vi "Vision Processing.vi"(4 "error in (no error)":errorcluster, 6 "CameraDevRef":T1) -> ()   [LabVIEW 2011]
uses:
  <vilib>/Rock Robotics/WPI/Camera/WPI_CameraDevRef.ctl
  Robot Global Data.vi
  <vilib>/vision/NI_Vision_Development_Module.lvlib
panel:
  in  "Max Distance for 1 hoop":dbl=8.0
  out "Raw Turret":dbl
  in  "Run Calculations":bool
  out "Target X Coord":dbl
  out "Target Distance":dbl
  out "Target Y Coord":dbl
  out "Distance Array":dbl[](array[numeric])
  in  "Scaler":dbl=0.85
  in  "Lower Speed Limit":dbl=0.05
  out "Number of Rectangles Visible":dbl
  out "Y Position Array":dbl[](array[numeric])
  out "X Position Array":dbl[](array[numeric])
  in  "View":bool
  out "Target Info":T2(array[cluster])
  in  "Area Size Limit":i32=444
  in  "Particle Count Limit":i32=8
  in  "Score Limits":T3={"Rect Coverage"=76.0, "Aspect Ratio"=40.0, "X Edge Strength"=40.0, "Y Edge Strength"=60.0}
  in  "Processing":enum32{"Color", "Intensity", "Intensity Open"}(tab)=enum."Intensity"
  in  "Luminance":i32=255
  in  "Saturation":i32=255
  in  "Hue":i32(knob)=65 scale=0.0..255.0
  in  "Margins":cluster{"Hue":i32, "Sat":i32, "Lum":i32}={"Hue"=20, "Sat"=27, "Lum"=30} {"Sat" scale=0.0..40.0; "Lum" scale=0.0..40.0; "Hue" scale=0.0..40.0}
  in  "Range":cluster{"Lower value":sgl, "Upper value":sgl}={"Lower value"=107.17391, "Upper value"=255.0} {"Lower value" scale=0.0..255.0; "Upper value" scale=0.0..255.0}
  in  "Range":cluster{"Lower value":sgl, "Upper value":sgl}={"Lower value"=123.804344, "Upper value"=255.0} {"Lower value" scale=0.0..255.0; "Upper value" scale=0.0..255.0}
  in  "View":bool
  out "Processed Image":T4(plugin-control)
  out "Original Image":T4(plugin-control)
  # "Instructions:\nProcessing the reflective tape that is illuminated by a ring light can be based\non color or light intensity.\nParticles within the image are scored by rectangle coverage, aspect ratio, and\nfor being hollow with a bold edge. A particle is considered a target if all scores\nare above the score limits. Particles can be annotated -- surrounded by\na rectangle and scores drawn to the left .\nTo control the number of particles being scored, use the count limit and the size\nlimit."
  # "(in)"
  # "To debug, Enable using the View button.\nFor color processing, you can click in the image to select the color for processing."
  # "Enable by clicking the View button.\nGreen scores are above the limit, orange are below. Inner/outer rect\nindicates all passed."
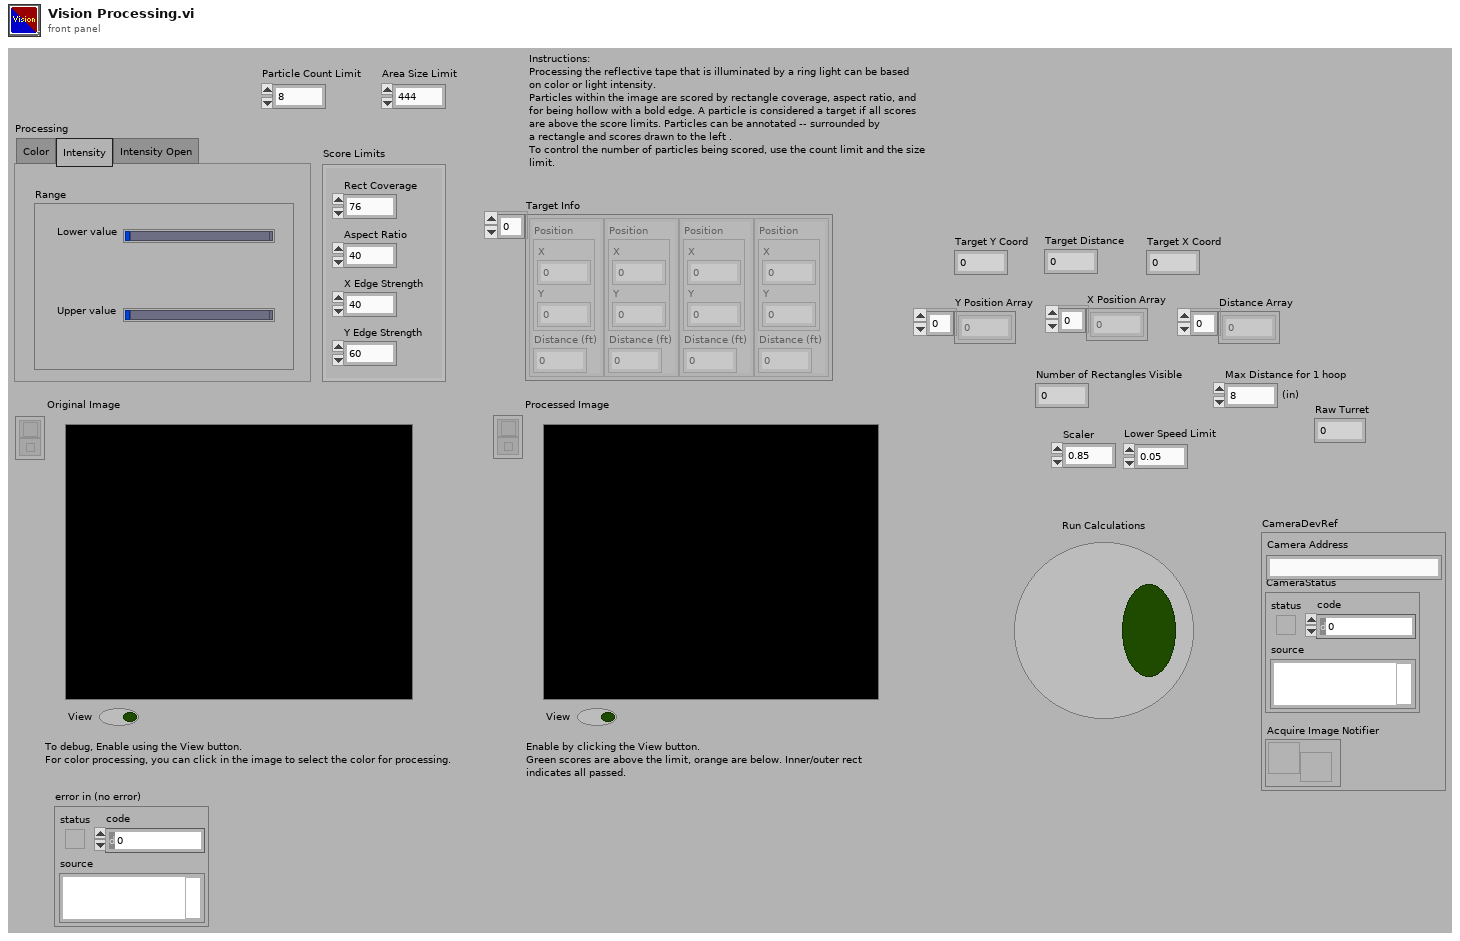
[diagram p1: front panel]
types:
  T1 = typedef "WPI_CameraDevRef.ctl" = cluster{"Camera Address":string, "CameraStatus":errorcluster, "Acquire Image Notifier":refnum<notifier>}
  T2 = cluster{"Position":cluster{"X":dbl, "Y":dbl}, "Distance (ft)":dbl}[]
  T3 = cluster{"Rect Coverage":dbl, "Aspect Ratio":dbl, "X Edge Strength":dbl, "Y Edge Strength":dbl}
  T4 = typedef "IMAQ Image.ctl" = refnum<image>
  T5 = typedef "Image Type" = u32
  T6 = enum32{"AutoM", "Close", "Dilate", "Erode", "Gradient", "Gradient out", "Gradient in", "Hit miss", "Open", "PClose", "POpen", "Thick", "Thin"}
  T7 = typedef "WPI_CameraImageSize.ctl" = enum16{"640x480", "320x240", "160x120"}
  T8 = cluster{"fps":i32, "compression":i32, "Image Size":T7}
  T9 = cluster{cluster{"Left":dbl, "Top":dbl, "Right":dbl, "Bottom":dbl}, dbl[]}[]
  T10 = cluster{"Left":dbl, "Top":dbl, "Right":dbl, "Bottom":dbl}
  T11 = cluster{"Target Center (-1 to 1)":cluster{"X":dbl, "Y":dbl}, "Distance (ft)":dbl}
  T12 = cluster{"Target Center (-1 to 1)":cluster{"X":dbl, "Y":dbl}, "Distance (ft)":dbl}[]
  T13 = typedef "WPI_JoystickDevRef.ctl" = cluster{"Device":T14}
  T14 = typedef "WPI_JoystickDeviceEnum.ctl" = enum16{"USB 1", "USB 2", "USB 3", "USB 4", "Kinect 1", "Kinect 2"}
  T15 = typedef "WPI_JoystickButtonState.ctl" = cluster{"Button 1":bool, "Button 2":bool, "Button 3":bool, "Button 4":bool, "Button 5":bool, "Button 6":bool, "Button 7":bool, "Button 8":bool, "Button 9":bool, "Button 10":bool, "Button 11":bool, "Button 12":bool}
  T16 = cluster{"axis 1 (x)":dbl, "axis 2 (y)":dbl, "axis 3 (throttle)":dbl, "axis 4":dbl, "axis 5":dbl, "axis 6":dbl}
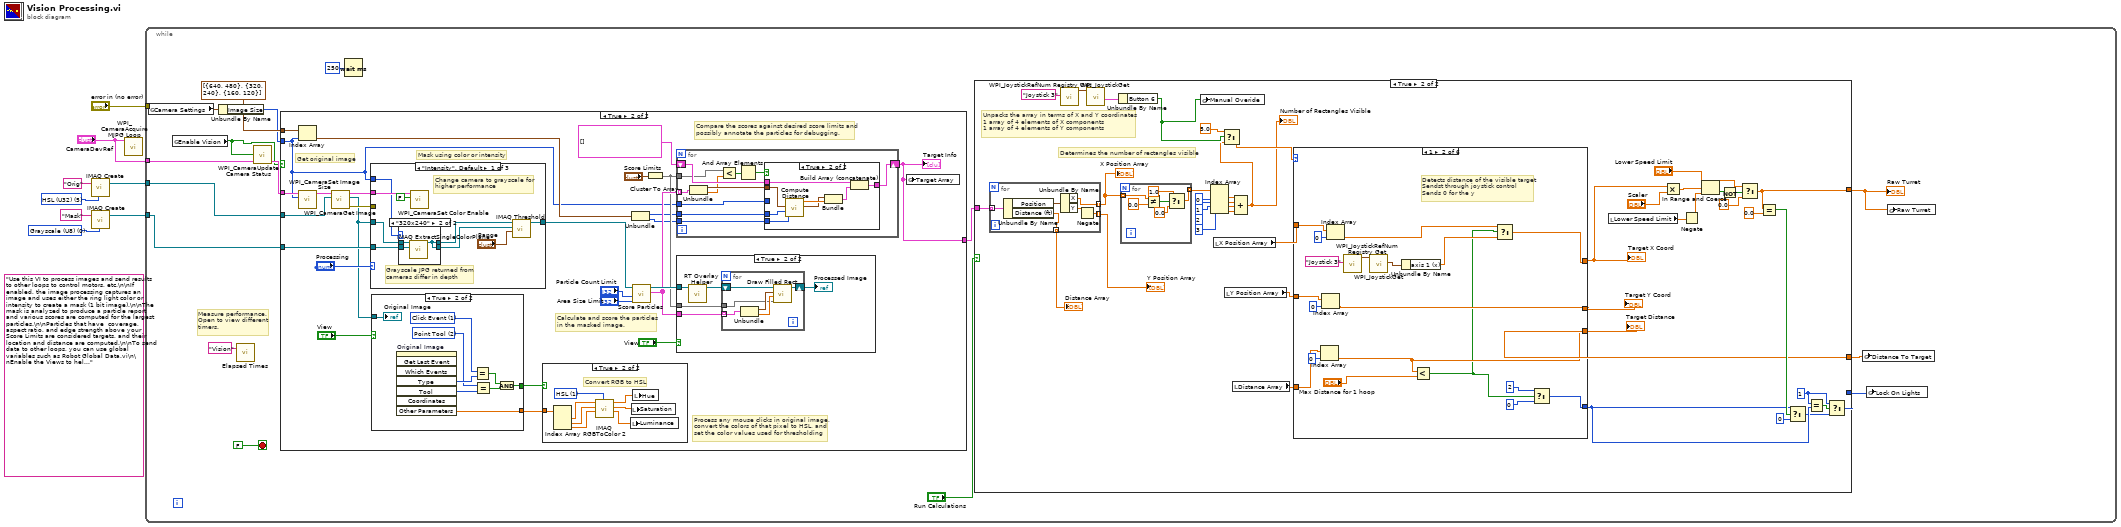
[diagram p0: block diagram]
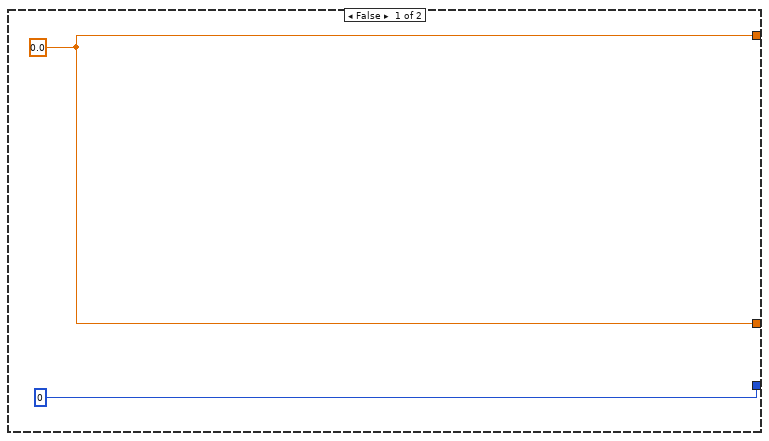
[diagram p2: hidden frame]
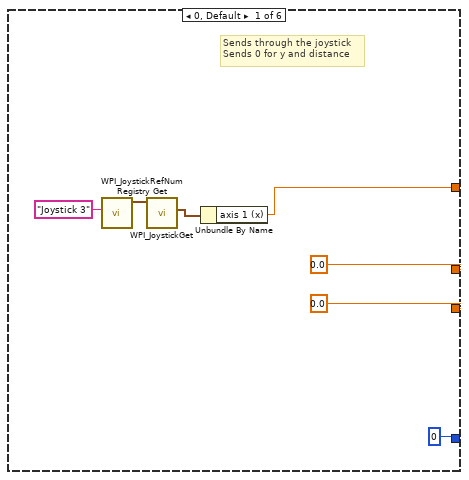
[diagram p3: hidden frame]
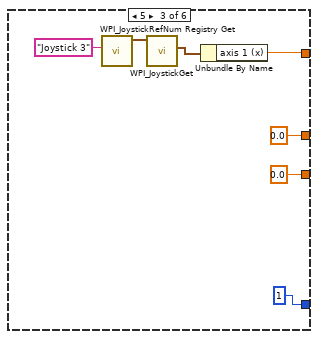
[diagram p4: hidden frame]
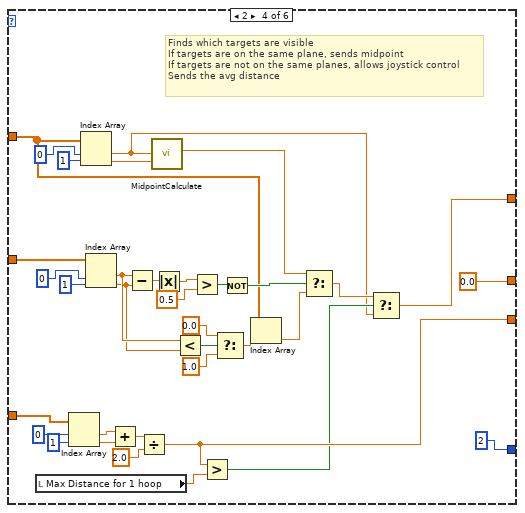
[diagram p5: hidden frame]
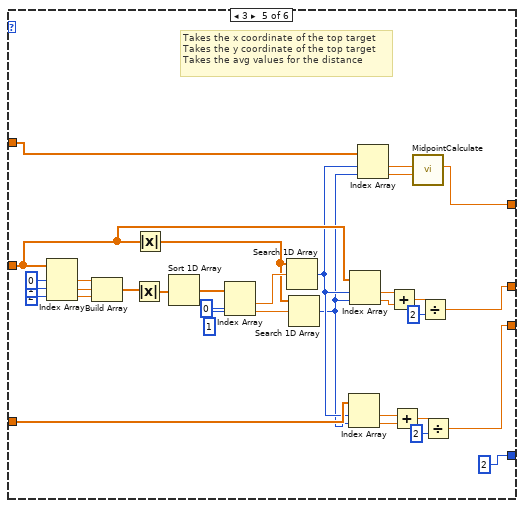
[diagram p6: hidden frame]
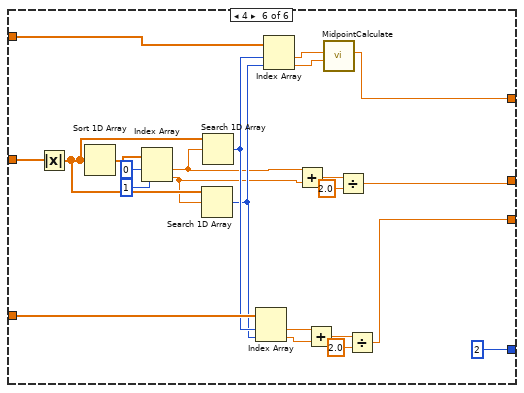
[diagram p7: hidden frame]
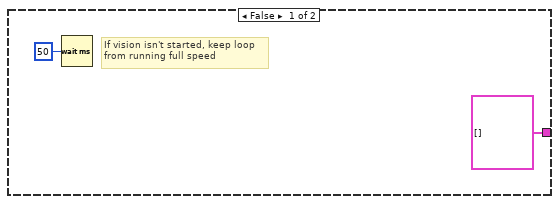
[diagram p8: hidden frame]
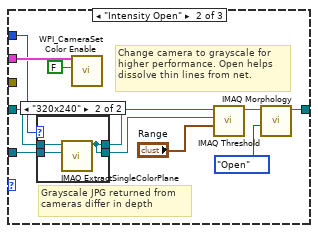
[diagram p11: hidden frame]
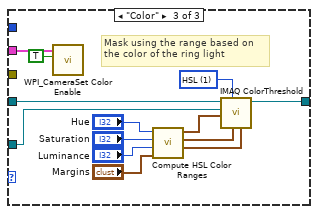
[diagram p13: hidden frame]
diagram:
  w3 = T5 0 items=["Grayscale (U8)", "Grayscale (I16)", "Grayscale (SGL)", "Complex (CSG)", "RGB (U32)", "HSL (U32)", "RGB (U64)", "Grayscale (U16)"] ("Image Type")
  (unwired) "Use this VI to process images and send results to other loops to control motors, etc.\n\nIf enabled, the image processing captures an image and uses either the ring light color or intensity to create a mask (1 bit image).\n\nThe mask is analyzed to produce a particle report and various scores are computed for the largest particles.\n\nParticles that have  coverage, aspect ratio, and edge strength above your Score Limits are considered targets, and their location and distance are computed.\n\nTo send data to other loops, you can use global variables such as Robot Global Data.vi\n\nEnable the Views to help debug color settings. Disable the View to speed up processing."
  w7 = T5 5 items=["Grayscale (U8)", "Grayscale (I16)", "Grayscale (SGL)", "Complex (CSG)", "RGB (U32)", "HSL (U32)", "RGB (U64)", "Grayscale (U16)"] ("Image Type")
  n1 = call "IMAQ Create"("Image Name"="Orig", "Image Type"=w7) -> ("New Image"=w6:T4)  [unwired: 2 in, 2 out]
  n2 = call "IMAQ Create"("Image Name"="Mask", "Image Type"=w3) -> ("New Image"=w1:T4)  [unwired: 2 in, 2 out]
  n3 = call <vilib>:"WPI_CameraAcquire MJPG Loop.vi"("CameraDevRef"="CameraDevRef") -> ()  [unwired: 11 in]
  n4 = while {
    tunnel: w6 -> [w23]
    tunnel: "CameraDevRef" -> [w22]
    tunnel: "error in (no error)" -> [_]
    tunnel: w1 -> [w18]
    stop <- FALSE stop-if-true
    # "Measure performance.\nOpen to view different\ntimers."
    n5 = global read "Robot Global Data.vi" "Camera Settings"() -> (w16:T8)
    n6 = global read "Robot Global Data.vi" "Enable Vision"() -> (w20:bool)
    n7 = Unbundle By Name(w16) -> ("Image Size"=w15:T7)
    n8 = call "Elapsed Times.vi"("Call Name"="Vision") -> ()  [unwired: 2 in, 1 out]
    n9 = call <vilib>:"WPI_CameraUpdate Camera Status.vi"("CameraDevRef In"=w22, "Enable Vision"=w20) -> ("CameraDevRef Out"=w21:T1)  [unwired: 3 in]
    n10 = case shown="True" w20 {
      tunnel: w23 -> [_ w224]
      tunnel: w21 -> [_ w220]
      tunnel: w18 -> [_ w211]
      tunnel: cluster{i32, i32}[] [{640, 480}, {320, 240}, {160, 120}] -> [_ w215]
      tunnel: w15 -> [_ w208]
      tunnel: [T2 [] w209] -> w14
      frame False {
        # "If vision isn't started, keep loop\nfrom running full speed"
        n11 = Wait (ms)(milliseconds to wait=u32 50) -> ()  [unwired: 1 out]
      }
      frame True {
        # "Compare the scores against desired score limits and\npossibly annotate the particles for debugging."
        # "Process any mouse clicks in original image,\nconvert the colors of that pixel to HSL, and\nset the color values used for thresholding"
        # "Calculate and score the particles\nin the masked image."
        # "Mask using color or intensity"
        # "Get original image"
        n12 = call <vilib>:"WPI_CameraSet Image Size.vi"("Image Size"=w208, "CameraDevRef"=w220) -> ("CameraDevRef Out"=w221:T1)  [unwired: 8 in, 1 out]
        n13 = Index Array(array=w215, index=w208) -> (element=w212:cluster{i32, i32})
        n14 = call <vilib>:"WPI_CameraGet Image.vi"("Image"=w224, "CameraDevRef"=w221) -> ("error out"=w222:errorcluster, "Image Out"=w210:T4, "CameraDevRef Out"=w223:T1)  [unwired: 7 in]
        n15 = case shown="\"Intensity\", Default" "Processing" {
          tunnel: w210 -> [w246 w258 w284]
          tunnel: [w249 w263 w283] -> w218
          tunnel: w223 -> [w247 w261 w274]
          tunnel: w222 -> [_ _ _]
          tunnel: w211 -> [w245 w259 w272]
          tunnel: w208 -> [w244 w260 _]
          frame "Intensity", Default {
            # "Grayscale JPG returned from\ncameras differ in depth"
            # "Change camera to grayscale for\nhigher performance"
            n16 = case shown="\"320x240\"" w244 {
              tunnel: w246 -> [w252 w255]
              tunnel: w245 -> [w251 w254]
              tunnel: [w252 w253] -> w243
              tunnel: [w251 w253] -> w242
              frame "640x480", Default {
              }
              frame "320x240" {
                n17 = call "IMAQ ExtractSingleColorPlane"("Image Dst"=w254, "Image Src"=w255) -> ("Image Dst Out"=w253:T4)  [unwired: 8 in, 1 out]
              }
            }
            n18 = call <vilib>:"WPI_CameraSet Color Enable.vi"("Color Enabled"=FALSE, "CameraDevRef"=w247) -> ()  [unwired: 8 in, 2 out]
            n19 = call "IMAQ Threshold"("Range"="Range", "Image Dst"=w242, "Image Src"=w243) -> ("Image Dst Out"=w249:T4)  [unwired: 3 in, 5 out]
          }
          frame "Intensity Open" {
            # "Grayscale JPG returned from\ncameras differ in depth"
            # "Change camera to grayscale for\nhigher performance. Open helps\ndissolve thin lines from net."
            n20 = case shown="\"320x240\"" w260 {
              tunnel: w258 -> [w268 w271]
              tunnel: w259 -> [w267 w270]
              tunnel: [w268 w269] -> w257
              tunnel: [w267 w269] -> w256
              frame "640x480", Default {
              }
              frame "320x240" {
                n21 = call "IMAQ ExtractSingleColorPlane"("Image Dst"=w270, "Image Src"=w271) -> ("Image Dst Out"=w269:T4)  [unwired: 8 in, 1 out]
              }
            }
            n22 = call <vilib>:"WPI_CameraSet Color Enable.vi"("Color Enabled"=FALSE, "CameraDevRef"=w261) -> ()  [unwired: 8 in, 2 out]
            n23 = call "IMAQ Threshold"("Range"="Range", "Image Dst"=w256, "Image Src"=w257) -> ("Image Dst Out"=w264:T4)  [unwired: 3 in, 5 out]
            n24 = call "IMAQ Morphology"("Operation"=T6."Open", "Image Src"=w264) -> ("Image Dst Out"=w263:T4)  [unwired: 8 in, 1 out]
          }
          frame "Color" {
            w282 = u16 1 items=["RGB", "HSL", "HSV", "HSI"] ("Color Mode")
            # "Mask using the range based on\nthe color of the ring light"
            n25 = call <vilib>:"WPI_CameraSet Color Enable.vi"("Color Enabled"=TRUE, "CameraDevRef"=w274) -> ()  [unwired: 8 in, 2 out]
            n26 = call "Compute HSL Color Ranges.vi"("Margins"="Margins", "Luminance"="Luminance", "Saturation"="Saturation", "Hue"="Hue") -> ("Lum Range"=w279:cluster{i32, i32}, "Sat Range"=w280:cluster{i32, i32}, "Hue Range"=w281:cluster{i32, i32})  [unwired: 5 in]
            n27 = call "IMAQ ColorThreshold"("Blue or Luma or Val or Inten Range"=w279, "Green or Sat Range"=w280, "Color Mode"=w282, "Red or Hue Range"=w281, "Image Dst"=w272, "Image Src"=w284) -> ("Image Dst Out"=w283:T4)  [unwired: 4 in, 1 out]
          }
        }
        n28 = case shown="True" "View" {
          tunnel: w210 -> [_ w304]
          tunnel: [_ w299] -> w217
          tunnel: [_ w296] -> w216
          frame False {
          }
          frame True {
            w297 = 2 items=["None", "Selection Tool", "Point Tool", "Line Tool", "Rectangle Tool", "Oval Tool", "Polygon Tool", "ClosedFreehandTool", "Annulus Tool", "Rotated Rectangle Tool", "Zoom Tool", "Pan Tool", "Polyline Tool", "Freehand Tool"] ("Tool")
            w298 = 1 items=["No Event"=0, "Click Event"=1, "Draw Event"=2, "Size Event"=4, "Scroll Event"=5, "Double Click Event"=8] ("Type")
            n29 = invoke on="Original Image" class="ImageControl" method="Get Last Event"() -> ("Type"=w300:i32, "Tool"=w303:i32, "Other Parameters"=w296:sgl[])  [unwired: 8 in, 5 out]
            n30 = Equal?(x=w298, y=w300) -> (x = y?=w301:bool)
            n31 = Equal?(x=w297, y=w303) -> (x = y?=w302:bool)
            n32 = And(x=w301, y=w302) -> (x .and. y?=w299:bool)
            "Original Image" <- w304
          }
        }
        n33 = case shown="True" w217 {
          tunnel: w216 -> [_ w241]
          frame False {
          }
          frame True {
            w240 = u16 1 items=["RGB", "HSL", "HSV", "HSI", "CIE L*a*b*", "CIE XYZ"] ("Color Mode")
            # "Convert RGB to HSL"
            n34 = Index Array(array=w241) -> (element #1=w239:sgl, element #2=w237:sgl, element #3=w235:sgl)  [unwired: 3 in]
            n35 = call "IMAQ RGBToColor 2"("Color Mode"=w240, "Blue value"=w235, "Green value"=w237, "Red value"=w239) -> ("Blue or Luma or Val or Inten or Z or b*value"=w234:dbl, "Green or Sat or Y or a* value"=w236:dbl, "Red or Hue or X or L* value"=w238:dbl)  [unwired: 4 in, 1 out]
            n36 = local write "Luminance"(w234) -> ()
            n37 = local write "Saturation"(w236) -> ()
            n38 = local write "Hue"(w238) -> ()
          }
        }
        n39 = Unbundle(w212) -> (w214:i32, w213:i32)
        n40 = call "Score Particles.vi"("Area Size Limit"="Area Size Limit", "Particle Count Limit"="Particle Count Limit", "Image Refnum in"=w218) -> ("Scored Particle Info"=w229:T9, "Image Refnum out"=w232:T4)  [unwired: 7 in]
        n41 = Cluster To Array(cluster="Score Limits") -> (array=w227:dbl[])
        n42 = for {
          shift-right: [w314] -> w209
          shift-left: T2 [] -> [w315]
          tunnel: w214 -> [w313]
          tunnel: w229 -> [w311] mode=indexing
          tunnel: w227 -> [w306]
          tunnel: w208 -> [w310]
          tunnel: w213 -> [w305]
          n43 = Unbundle(w311) -> (w312:T10, w307:dbl[])
          n44 = Less?(x=w306, y=w307) -> (x < y?=w309:bool[])
          n45 = And Array Elements(Boolean array=w309) -> (logical AND=w308:bool)
          n46 = case shown="True" w308 {
            tunnel: w315 -> [w316 w324]
            tunnel: [w316 w323] -> w314
            tunnel: w312 -> [_ w319]
            tunnel: w313 -> [_ w321]
            tunnel: w310 -> [_ _]
            tunnel: w305 -> [_ w318]
            frame False {
            }
            frame True {
              n47 = call "Compute Distance.vi"("Y Image Resolution"=w318, "X Image Resolution"=w321, "Bounding Box"=w319) -> ("Target Center (-1 to 1)"=w317:cluster{"X":dbl, "Y":dbl}, "Distance (ft)"=w320:dbl)  [unwired: 7 in]
              n48 = Bundle("Target Center (-1 to 1)"=w317, "Distance (ft)"=w320) -> (w322:T11)  [unwired: 1 in]
              n49 = Build Array (concatenate)(w324, w322) -> (w323:T12)
            }
          }
        }
        "Target Info" <- w209
        n50 = case shown="True" "View" {
          tunnel: w232 -> [_ w286]
          tunnel: w229 -> [_ w288]
          tunnel: w227 -> [_ w287]
          frame False {
          }
          frame True {
            n51 = call "RT Overlay Helper.vi"("Refnum in"=w286) -> ("Refnum out"=w289:T4)  [unwired: 10 in]
            n52 = for {
              shift-right: [w294] -> w285
              shift-left: w289 -> [w295]
              tunnel: w288 -> [w291] mode=indexing
              tunnel: w287 -> [w290]
              n53 = Unbundle(w291) -> (w292:T10, w293:dbl[])
              n54 = call "Draw Filled Rect.vi"("Limits"=w290, "Scores"=w293, "Bounding Box"=w292, "image in"=w295) -> ("image out"=w294:T4)  [unwired: 7 in]
            }
            "Processed Image" <- w285
          }
        }
        n55 = global write "Robot Global Data.vi" "Target Array"(w209) -> ()
      }
    }
    n56 = Wait (ms)(milliseconds to wait=u32 250) -> ()  [unwired: 1 out]
    n57 = case shown="True" "Run Calculations" {
      tunnel: w14 -> [_ w42]
      tunnel: [w25 w36] -> w11
      tunnel: [0 ("f") w33] -> w10
      tunnel: [w25 w28] -> w9
      frame False {
        w25 = 0.0 ("f")
      }
      frame True {
        w34 = 1 ("y")
        # "Determines the number of rectangles visible"
        # "Unpacks the array in terms of X and Y coordinates\n1 array of 4 elements of X components\n1 array of 4 elements of Y components"
        n58 = for {
          tunnel: [w203] -> w43 mode=indexing
          tunnel: [w204] -> w53 mode=indexing
          tunnel: w42 -> [w201] mode=indexing
          tunnel: [w200] -> w62 mode=indexing
          n59 = Unbundle By Name(w201) -> ("Position"=w205:cluster{"X":dbl, "Y":dbl}, "Distance (ft)"=w200:dbl)
          n60 = Unbundle By Name(w205) -> ("X"=w204:dbl, "Y"=w202:dbl)
          n61 = Negate(x=w202) -> (-x=w203:dbl)
        }
        "X Position Array" <- w53
        "Y Position Array" <- w43
        "Distance Array" <- w62
        n62 = call <vilib>:"WPI_JoystickRefNum Registry Get.vi"("refnum name"="Joystick 3") -> ("JoystickDevRef"=w40:T13)  [unwired: 9 in, 1 out]
        n63 = call <vilib>:"WPI_JoystickGet.vi"("JoystickDevRef"=w40) -> ("Buttons"=w38:T15)  [unwired: 4 in, 2 out]
        n64 = Unbundle By Name(w38) -> ("Button 6"=w37:bool)
        n65 = for {
          tunnel: w53 -> [w74] mode=indexing
          tunnel: [w70] -> w52 mode=indexing
          n66 = Not Equal?(x=w74, y=0.0) -> (x != y?=w73:bool)
          n67 = Select(t=1.0, s=w73, f=0.0) -> (s? t:f=w70:dbl)
        }
        n68 = global write "Robot Global Data.vi" "Manual Overide"(w37) -> ()
        n69 = Index Array(array=w52, index #1=0 ("index"), index #2=1 ("index"), index #3=2 ("index"), index #4=3 ("index")) -> (element #1=w50:dbl, element #2=w51:dbl, element #3=w49:dbl, element #4=w48:dbl)
        n70 = local read "X Position Array"() -> (w54:dbl[])
        n71 = local read "Y Position Array"() -> (w65:dbl[])
        n72 = local read "Distance Array"() -> (w66:dbl[])
        n73 = Compound Arithmetic op=ADD(w50, w51, w49, w48) -> (w27:dbl)
        "Number of Rectangles Visible" <- w27
        n74 = Select(t=5.0, s=w37, f=w27) -> (s? t:f=w68:dbl)
        n75 = case shown="1" w68 {
          tunnel: w54 -> [_ w98 _ w117 w160 w194]
          tunnel: [w77 w90 w103 w110 w157 w184] -> w64
          tunnel: [0.0 ("X") w87 0.0 ("X") 0.0 ("X") w161 w183] -> w63
          tunnel: [0.0 ("X") w94 0.0 ("X") w114 w145 w178] -> w28
          tunnel: w65 -> [_ w88 _ w141 w153 w199]
          tunnel: w66 -> [_ w101 _ w127 w148 w193]
          tunnel: [0 w83 1 2 2 2] -> w31
          frame 0, Default {
            # "Sends through the joystick\nSends 0 for y and distance"
            n76 = call <vilib>:"WPI_JoystickRefNum Registry Get.vi"("refnum name"="Joystick 3") -> ("JoystickDevRef"=w80:T13)  [unwired: 9 in, 1 out]
            n77 = call <vilib>:"WPI_JoystickGet.vi"("JoystickDevRef"=w80) -> ("Axes"=w78:T16)  [unwired: 4 in, 2 out]
            n78 = Unbundle By Name(w78) -> ("axis 1 (x)"=w77:dbl)
          }
          frame 1 {
            # "Detects distance of the visible target\nSendst through joystick control\nSends 0 for the y"
            n79 = Index Array(array=w101, index=0) -> (element=w94:dbl)
            n80 = Index Array(array=w88, index=0) -> (element=w87:dbl)
            n81 = Index Array(array=w98, index=0) -> (element=w92:dbl)
            n82 = call <vilib>:"WPI_JoystickRefNum Registry Get.vi"("refnum name"="Joystick 3") -> ("JoystickDevRef"=w97:T13)  [unwired: 9 in, 1 out]
            n83 = call <vilib>:"WPI_JoystickGet.vi"("JoystickDevRef"=w97) -> ("Axes"=w95:T16)  [unwired: 4 in, 2 out]
            n84 = Unbundle By Name(w95) -> ("axis 1 (x)"=w91:dbl)
            n85 = Less?(x=w94, y="Max Distance for 1 hoop") -> (x < y?=w85:bool)
            n86 = Select(t=w92, s=w85, f=w91) -> (s? t:f=w90:dbl)
            n87 = Select(t=2, s=w85, f=0) -> (s? t:f=w83:i32)
          }
          frame 5 {
            n88 = call <vilib>:"WPI_JoystickRefNum Registry Get.vi"("refnum name"="Joystick 3") -> ("JoystickDevRef"=w106:T13)  [unwired: 9 in, 1 out]
            n89 = call <vilib>:"WPI_JoystickGet.vi"("JoystickDevRef"=w106) -> ("Axes"=w104:T16)  [unwired: 4 in, 2 out]
            n90 = Unbundle By Name(w104) -> ("axis 1 (x)"=w103:dbl)
          }
          frame 2 {
            # "Finds which targets are visible\nIf targets are on the same plane, sends midpoint\nIf targets are not on the same planes, allows joystick control\nSends the avg distance"
            n91 = local read "Max Distance for 1 hoop"() -> (w113:dbl)
            n92 = Index Array(array=w127, index #1=0 ("index"), index #2=1 ("index")) -> (element #1=w126:dbl, element #2=w125:dbl)
            n93 = Index Array(array=w117, index #1=0 ("index"), index #2=1 ("index")) -> (element #1=w109:dbl, element #2=w131:dbl)
            n94 = Index Array(array=w141, index #1=0 ("index"), index #2=1 ("index")) -> (element #1=w123:dbl, element #2=w122:dbl)
            n95 = Add(x=w126, y=w125) -> (x+y=w130:dbl)
            n96 = Subtract(x=w123, y=w122) -> (x-y=w138:dbl)
            n97 = Divide(x=w130, y=2.0) -> (x/y=w114:dbl)
            n98 = call "MidpointCalculate.vi"("X2"=w131, "X1"=w109) -> ("Midpoint"=w133:dbl)  [unwired: 9 in]
            n99 = Absolute Value(x=w138) -> (abs(x)=w137:dbl)
            n100 = Less?(x=w123, y=w122) -> (x < y?=w121:bool)
            n101 = Greater?(x=w137, y=0.5) -> (0:w134:bool)
            n102 = Greater?(x=w114, y=w113) -> (0:w112:bool)
            n103 = Select(t=0.0, s=w121, f=1.0) -> (s? t:f=w118:dbl)
            n104 = Not(x=w134) -> (.not. x?=w135:bool)
            n105 = Index Array(array=w117, index=w118) -> (element=w116:dbl)
            n106 = Select(t=w133, s=w135, f=w116) -> (s? t:f=w111:dbl)
            n107 = Select(t=w111, s=w112, f=w109) -> (s? t:f=w110:dbl)
          }
          frame 3 {
            # "Takes the x coordinate of the top target\nTakes the y coordinate of the top target\nTakes the avg values for the distance"
            n108 = Index Array(array=w153, index #1=0 ("index"), index #2=1 ("index"), index #3=2 ("index")) -> (element #1=w173:dbl, element #2=w172:dbl, element #3=w171:dbl)
            n109 = Build Array(w173, w172, w171) -> (w170:dbl[])
            n110 = Absolute Value(x=w170) -> (abs(x)=w164:dbl[])
            n111 = Absolute Value(x=w153) -> (abs(x)=w156:dbl[])
            n112 = Sort 1D Array(array=w164) -> (sorted array=w169:dbl[])
            n113 = Index Array(array=w169, index #1=0 ("index"), index #2=1 ("index")) -> (element #1=w165:dbl, element #2=w166:dbl)
            n114 = Search 1D Array(1D array=w156, element=w165) -> (index of element=w147:i32)  [unwired: 1 in]
            n115 = Search 1D Array(1D array=w156, element=w166) -> (index of element=w146:i32)  [unwired: 1 in]
            n116 = Index Array(array=w148, index #1=w147, index #2=w146) -> (element #1=w150:dbl, element #2=w149:dbl)
            n117 = Index Array(array=w153, index #1=w147, index #2=w146) -> (element #1=w155:dbl, element #2=w154:dbl)
            n118 = Index Array(array=w160, index #1=w147, index #2=w146) -> (element #1=w159:dbl, element #2=w158:dbl)
            n119 = Add(x=w155, y=w154) -> (x+y=w163:dbl)
            n120 = Add(x=w150, y=w149) -> (x+y=w151:dbl)
            n121 = call "MidpointCalculate.vi"("X2"=w158, "X1"=w159) -> ("Midpoint"=w157:dbl)  [unwired: 9 in]
            n122 = Divide(x=w163, y=2) -> (x/y=w161:dbl)
            n123 = Divide(x=w151, y=2) -> (x/y=w145:dbl)
          }
          frame 4 {
            n124 = Absolute Value(x=w199) -> (abs(x)=w195:dbl[])
            n125 = Sort 1D Array(array=w195) -> (sorted array=w198:dbl[])
            n126 = Index Array(array=w198, index #1=0 ("index"), index #2=1 ("index")) -> (element #1=w190:dbl, element #2=w189:dbl)
            n127 = Search 1D Array(1D array=w195, element=w189) -> (index of element=w191:i32)  [unwired: 1 in]
            n128 = Search 1D Array(1D array=w195, element=w190) -> (index of element=w192:i32)  [unwired: 1 in]
            n129 = Index Array(array=w193, index #1=w192, index #2=w191) -> (element #1=w180:dbl, element #2=w179:dbl)
            n130 = Index Array(array=w194, index #1=w192, index #2=w191) -> (element #1=w186:dbl, element #2=w185:dbl)
            n131 = Add(x=w190, y=w189) -> (x+y=w188:dbl)
            n132 = Add(x=w180, y=w179) -> (x+y=w181:dbl)
            n133 = call "MidpointCalculate.vi"("X2"=w185, "X1"=w186) -> ("Midpoint"=w184:dbl)  [unwired: 9 in]
            n134 = Divide(x=w188, y=2.0) -> (x/y=w183:dbl)
            n135 = Divide(x=w181, y=2.0) -> (x/y=w178:dbl)
          }
        }
        "Target Y Coord" <- w63
        "Target Distance" <- w28
        "Target X Coord" <- w64
        n136 = local read "Lower Speed Limit"() -> (w56:dbl)
        n137 = Multiply(x=w64, y="Scaler") -> (x*y=w61:dbl)
        n138 = Negate(x=w56) -> (-x=w57:dbl)
        n139 = In Range and Coerce(upper limit="Lower Speed Limit", x=w61, lower limit=w57) -> (In Range?=w58:bool)  [unwired: 1 out]
        n140 = Not(x=w58) -> (.not. x?=w59:bool)
        n141 = Select(t=w61, s=w59, f=0.0) -> (s? t:f=w36:dbl)
        n142 = Equal?(x=w36, y=0.0) -> (x = y?=w32:bool)
        n143 = Select(t=w31, s=w32, f=0) -> (s? t:f=w29:i32)
        n144 = Equal?(x=w34, y=w31) -> (x = y?=w35:bool)
        n145 = Select(t=w34, s=w35, f=w29) -> (s? t:f=w33:i32)
      }
    }
    "Raw Turret" <- w11
    n146 = global write "Robot Global Data.vi" "Distance To Target"(w9) -> ()
    n147 = global write "Robot Global Data.vi" "Lock On Lights"(w10) -> ()
    n148 = global write "Robot Global Data.vi" "Raw Turret"(w11) -> ()
  }
